vi "20211029_05.vi"() -> ()   [LabVIEW 2019]
uses:
  <vilib>/numeric/Random Number (Range) U64.vi
  <vilib>/numeric/sub_Random U32.vi
panel:
  out "Numeric":u64
  out "Array":u64[](array[numeric])
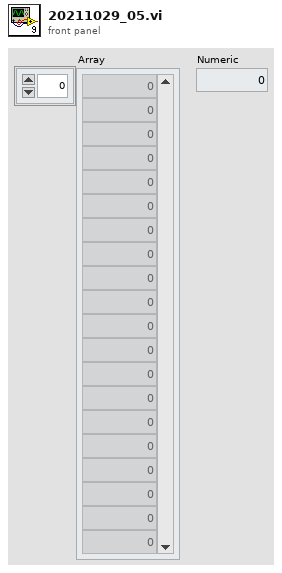
[diagram p1: front panel]
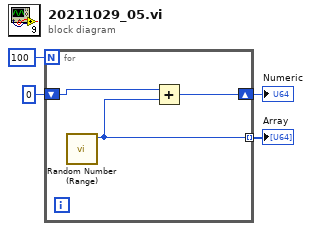
[diagram p0: block diagram]
diagram:
  n1 = for {
    N: 100 -> [_]
    shift-right: [w7] -> w1
    shift-left: u64 0 -> [w6]
    tunnel: [w5] -> w2 mode=indexing
    n2 = call-poly <vilib>:"Random Number (Range).vi"() -> ("number"=w5:u64)  [unwired: 11 in]
    n3 = Add(x=w6, y=w5) -> (x+y=w7:u64)
  }
  "Array" <- w2
  "Numeric" <- w1
